vi "StartTestSuite.vi"(8 "error in (no error)":errorcluster, 10 "TestSuite":refnum<class "TestSuite.lvclass">, 11 "TestResult in":refnum<class "TestResult.lvclass">) -> (0 "error out":errorcluster, 3 "TestResult out":refnum<class "TestResult.lvclass">)   [LabVIEW 2019, in "TestResult.lvclass"]
uses:
  TestResult.lvclass
  TestListener/TestListener.lvclass
  TestSuite/TestSuite.lvclass
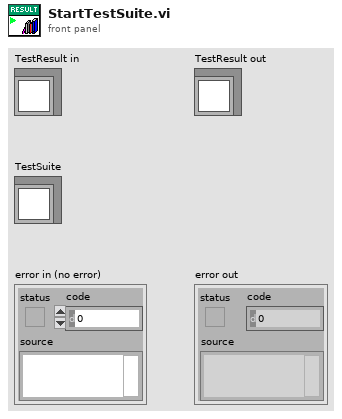
[diagram p1: front panel]
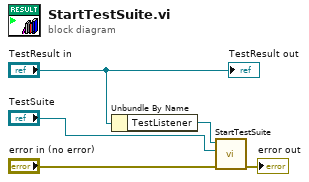
[diagram p0: block diagram]
diagram:
  n1 = Unbundle By Name("TestResult in") -> ("TestListener"=w4:refnum<class "TestListener.lvclass">)
  n2 = call-dynamic "StartTestSuite.vi"("error in (no error)"="error in (no error)", "TestSuite"="TestSuite", "TestListener in"=w4) -> ("error out"=→"error out":errorcluster)  [unwired: 7 in, 1 out]
  "TestResult out" <- "TestResult in"
